vi "Init Controls.vi"(8 "Inputs":refnum<vi>[][](array[refnum]), 9 "Labels":refnum<vi>[][](array[refnum]), 10 "Outputs":refnum<vi>[][](array[refnum]), 11 "MUX Config":T1[](array[typedef])=[{"Outputs"=[{"Desk Left", 2817882}, {"Desk Center", 2817882}, {"Desk Right", 2817882}, {"Bench Left", 12492800}, {"Bench Right", 12492800}, {"F", 7171459}, {"G", 7171459}, {"Mux Out", 16746514}], "Inputs"=[{"Desktop 1", 16448250}, {"Desktop 2", 16448250}, {"Desktop 3", 16448250}, {"Dock 1", 7078143}, {"Dock 2", 7078143}, {"Dock 3", 7078143}, {"Red HDMI", 16727100}, {"Mux In", 16750705}]}, {"Outputs"=[{"TV", 16775513}, {"", 0}, {"", 0}, {"", 0}, {"", 0}, {"", 0}, {"HD60S Capture", 44252}, {"Mux Out", 16750705}], "Inputs"=[{"Blu-ray", 9567230}, {"2", 0}, {"3", 0}, {"4", 0}, {"Consoles", 16711776}, {"5", 0}, {"Blue HDMI", 2768895}, {"Mux In", 16746514}]}]) -> ()   [LabVIEW 2022 SP3, in "TouchControl.lvlib" / "MuxPanel.lvclass"]
uses:
  MuxPanel.lvclass
  MUX Config.ctl
  MUX Element.ctl
  MuxPanel.lvclass/MuxPanel.ctl
  TouchControl.lvlib
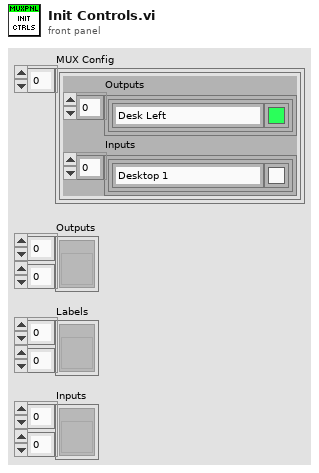
[diagram p1: front panel]
types:
  T1 = typedef "TouchControl.lvlib/MUX Config.ctl" = cluster{"Outputs":T2[], "Inputs":T2[]}
  T2 = typedef "TouchControl.lvlib/MUX Element.ctl" = cluster{string, u32}
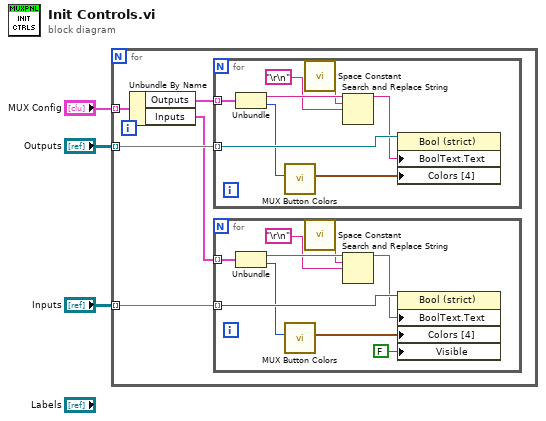
[diagram p0: block diagram]
diagram:
  n1 = for {
    tunnel: "Outputs" -> [w8] mode=indexing
    tunnel: "MUX Config" -> [w7] mode=indexing
    tunnel: "Inputs" -> [w4] mode=indexing
    n2 = Unbundle By Name(w7) -> ("Outputs"=w6:T2[], "Inputs"=w5:T2[])
    n3 = for {
      tunnel: w8 -> [w25] mode=indexing
      tunnel: w6 -> [w23] mode=indexing
      n4 = Unbundle(w23) -> (w21:string, w22:u32)
      n5 = call "MUX Button Colors.vi"("Color"=w22) -> ("MUX Button Colors"=w24:cluster{"Shadow":u32, "Shadow":u32}[])  [unwired: 10 in]
      n6 = call <vilib>:"Space Constant.vi"() -> ("String"=w20:string)
      n7 = Search and Replace String(input string=w21, search string=w20, replace string="\r\n") -> (result string=w19:string)  [unwired: 5 in, 3 out]
      n8 = property class="Bool (strict)"(reference=w25, "BoolText.Text"=w19, "Colors [4]"=w24) -> ()  [unwired: 1 in, 2 out]
    }
    n9 = for {
      tunnel: w4 -> [w17] mode=indexing
      tunnel: w5 -> [w15] mode=indexing
      n10 = Unbundle(w15) -> (w13:string, w14:u32)
      n11 = call "MUX Button Colors.vi"("Color"=w14) -> ("MUX Button Colors"=w16:cluster{"Shadow":u32, "Shadow":u32}[])  [unwired: 10 in]
      n12 = call <vilib>:"Space Constant.vi"() -> ("String"=w12:string)
      n13 = Search and Replace String(input string=w13, search string=w12, replace string="\r\n") -> (result string=w11:string)  [unwired: 5 in, 3 out]
      n14 = property class="Bool (strict)"(reference=w17, "BoolText.Text"=w11, "Colors [4]"=w16, "Visible"=FALSE) -> ()  [unwired: 1 in, 2 out]
    }
  }
